vi "2020_day08 (subVI replace nop_jmp).vi"(7 "Mode":enum16{"jmp to nop", "nop to jmp"}(ring), 9 "Start Line In":i32, 11 "Array In":string[](array[string])) -> (1 "Start Line Out":i32, 3 "Array Out":string[](array[string]), 4 "End of Replacement Reached?":bool)   [LabVIEW 2021]
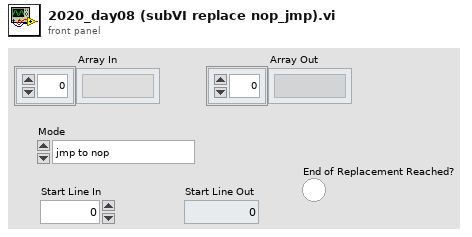
[diagram p1: front panel]
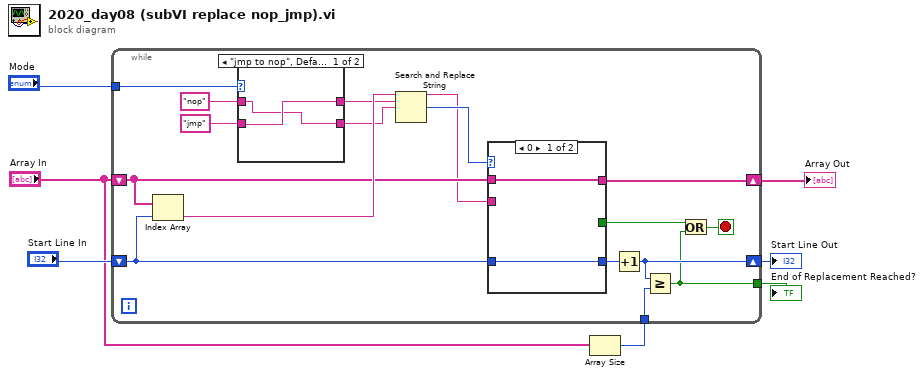
[diagram p0: block diagram]
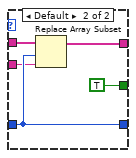
[diagram p2: hidden frame]
diagram:
  n1 = Array Size(array="Array In") -> (size(s)=w2:i32)
  n2 = while {
    tunnel: "Mode" -> [w24]
    shift-right: [w11] -> w4
    shift-left: "Start Line In" -> [w16]
    shift-right: [w13] -> w5
    shift-left: "Array In" -> [w18]
    tunnel: w2 -> [w10]
    tunnel: [w8] -> w1
    stop <- w9 stop-if-true
    n3 = Index Array(array=w18, index=w16) -> (element=w23:string)
    n4 = case shown="\"jmp to nop\", Default" w24 {
      tunnel: "nop" -> [w32 w35]
      tunnel: [w33 w35] -> w21
      tunnel: [w32 w34] -> w20
      tunnel: "jmp" -> [w33 w34]
      frame "jmp to nop", Default {
      }
      frame "nop to jmp" {
      }
    }
    n5 = Search and Replace String(input string=w23, search string=w21, replace string=w20) -> (result string=w12:string, number of replacements=w17:i32)  [unwired: 5 in, 2 out]
    n6 = case shown="0" w17 {
      tunnel: w18 -> [w25 w31]
      tunnel: w16 -> [w26 w30]
      tunnel: [w26 w30] -> w15
      tunnel: [_ TRUE] -> w14
      tunnel: [w25 w28] -> w13
      tunnel: w12 -> [_ w27]
      frame 0 {
      }
      frame Default {
        n7 = Replace Array Subset(array=w31, new element=w27, index=w30) -> (w28:string[])
      }
    }
    n8 = Increment(x=w15) -> (x+1=w11:i32)
    n9 = Greater Or Equal?(x=w11, y=w10) -> (x >= y?=w8:bool)
    n10 = Or(x=w14, y=w8) -> (x .or. y?=w9:bool)
  }
  "Array Out" <- w5
  "Start Line Out" <- w4
  "End of Replacement Reached?" <- w1
